vi "Galil Read Variables.vi"(8 "error in (no error)":errorcluster, 10 "Var Names":string[](array[string]), 11 "Automation Refnum in":refnum<k7>) -> (0 "error out":errorcluster, 1 "Valid?":bool, 2 "Values":dbl[](array[numeric]), 3 "Automation Refnum out":refnum<k7>)   [LabVIEW 2013]
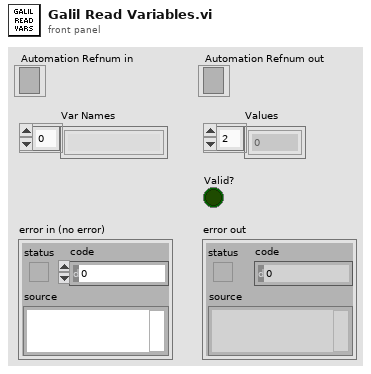
[diagram p1: front panel]
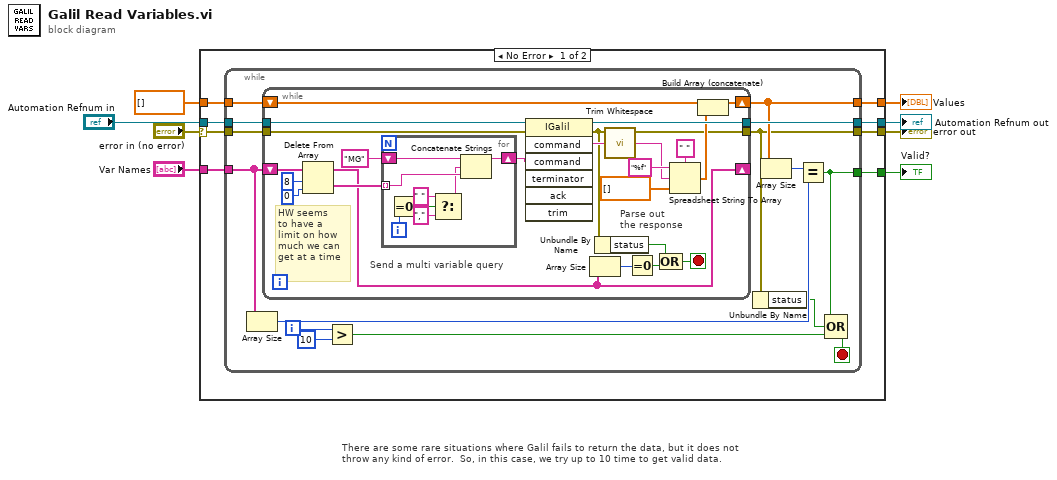
[diagram p0: block diagram]
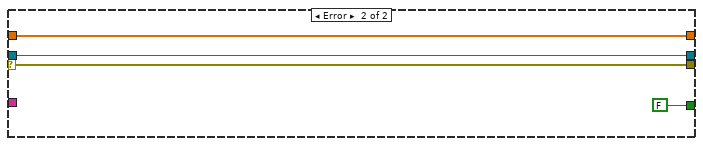
[diagram p2: hidden frame]
diagram:
  # "There are some rare situations where Galil fails to return the data, but it does not\nthrow any kind of error.  So, in this case, we try up to 10 time to get valid data."
  n1 = case shown="No Error" "error in (no error)" {
    selector: "error in (no error)" -> [w9 w64]
    tunnel: [w16 w64] -> w1
    tunnel: [w15 w65] -> w2
    tunnel: "Automation Refnum in" -> [w14 w65]
    tunnel: dbl[] [] ("array type (2D Dbl)") -> [w13 w66]
    tunnel: "Var Names" -> [w12 _]
    tunnel: [w11 w66] -> w5
    tunnel: [w10 FALSE] -> w6
    frame No Error {
      n2 = while {
        tunnel: w9 -> [w31]
        tunnel: [w18] -> w16
        tunnel: [w30] -> w15
        tunnel: w14 -> [w29]
        tunnel: w13 -> [w28]
        tunnel: w12 -> [w27]
        tunnel: [w26] -> w11
        tunnel: [w23] -> w10
        i -> [w21]
        stop <- w22 stop-if-true
        n3 = Array Size(array=w27) -> (size(s)=w24:i32)
        n4 = while {
          tunnel: w31 -> [w54]
          tunnel: [w34] -> w18
          tunnel: [w53] -> w30
          tunnel: w29 -> [w52]
          shift-right: [w41] -> _
          shift-left: w27 -> [w44]
          shift-right: [w37] -> w26
          shift-left: w28 -> [w38]
          stop <- w33 stop-if-true
          # "HW seems\nto have a\nlimit on how\nmuch we can\nget at a time"
          # "Parse out \nthe response"
          # "Send a multi variable query"
          n5 = Delete From Array(array=w44, length=8 ("y"), index=0) -> (deleted portion=w43:string[], array with subset deleted=w41:string[])
          n6 = for {
            tunnel: w43 -> [w61] mode=indexing
            shift-right: [w60] -> w50
            shift-left: "MG" ("command") -> [w62]
            i -> [w59]
            n7 = Equal To 0?(x=w59) -> (x = 0?=w58:bool)
            n8 = Select(t=" " ("command"), s=w58, f="," ("command")) -> (s? t:f=w57:string)
            n9 = Concatenate Strings(w62, w57, w61) -> (w60:string)
          }
          n10 = invoke class="IGalil" method="command"(reference=w52, error in=w54, "command"=w50) -> (reference out=w53:refnum<k7>, error out=w34:errorcluster, "command"=w49:string)  [unwired: 4 in, 4 out]
          n11 = Array Size(array=w41) -> (size(s)=w40:i32)
          n12 = Unbundle By Name(w34) -> ("status"=w32:bool)
          n13 = call <vilib>:"Trim Whitespace.vi"("string"=w49) -> ("trimmed string"=w45:string)  [unwired: 1 in]
          n14 = Equal To 0?(x=w40) -> (x = 0?=w39:bool)
          n15 = Compound Arithmetic op=OR(w32, w39) -> (w33:bool)
          n16 = Spreadsheet String To Array(delimiter (Tab)=" ", format string="%f", spreadsheet string=w45, array type (2D Dbl)=dbl[] []) -> (array=w36:dbl[])
          n17 = Build Array (concatenate)(w38, w36) -> (w37:dbl[])
        }
        n18 = Greater?(x=w21, y=10) -> (0:w19:bool)
        n19 = Unbundle By Name(w18) -> ("status"=w17:bool)
        n20 = Array Size(array=w26) -> (size(s)=w25:i32)
        n21 = Equal?(x=w25, y=w24) -> (x = y?=w23:bool)
        n22 = Compound Arithmetic op=OR(w23, w17, w19) -> (w22:bool)
      }
    }
    frame Error {
    }
  }
  "Automation Refnum out" <- w2
  "error out" <- w1
  "Values" <- w5
  "Valid?" <- w6
